vi "Function Set.vi"(6 "chip select  (1st chip)":enum16{"1st chip", "2nd chip"}(ring), 8 "error in (no error)":errorcluster, 10 "function set cmd code":u8, 11 "LCD in":u32) -> (0 "error out":errorcluster, 3 "LCD out":u32)   [LabVIEW 2015, in "HD44780 FPGA.lvlib"]
uses:
  <vilib>/EmbeddedDisplay/Hitachi HD44780/FPGA/HD44780 FPGA.lvlib
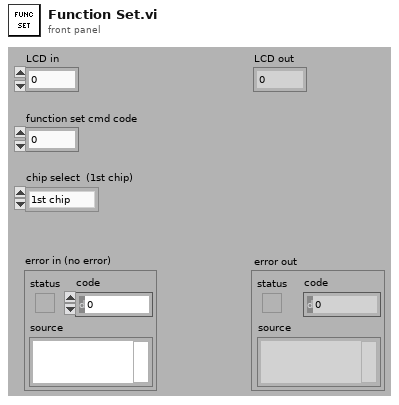
[diagram p1: front panel]
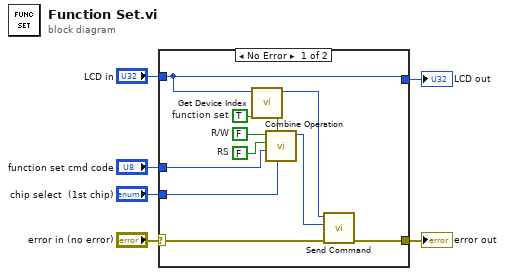
[diagram p0: block diagram]
diagram:
  n1 = case shown="No Error" "error in (no error)" {
    selector: "error in (no error)" -> [w12 w18]
    tunnel: "LCD in" -> [w7 w17]
    tunnel: [w7 w17] -> w5
    tunnel: [w16 w18] -> w4
    tunnel: "function set cmd code" -> [w9 _]
    tunnel: "chip select  (1st chip)" -> [w10 _]
    frame No Error {
      w13 = FALSE  # RS
      w14 = TRUE  # function set
      w15 = FALSE  # R/W
      n2 = call <vilib>:"Get Device Index.vi"("LCD in"=w7) -> ("device index"=w8:i8)  [unwired: 10 in]
      n3 = call <vilib>:"Combine Operation.vi"("chip select  (1st chip)"=w10, "function set (F)"=w14, "cmd/data (0)"=w9, "RS"=w13, "R/W"=w15) -> ("output"=w11:u32)  [unwired: 6 in]
      n4 = call <vilib>:"Send Command.vi"("error in (no error)"=w12, "operation"=w11, "device index"=w8) -> ("error out"=w16:errorcluster)  [unwired: 6 in, 2 out]
    }
    frame Error {
    }
  }
  "LCD out" <- w5
  "error out" <- w4
